vi "getWSIOpenCVIP.vi"(3 "File Path":path=path "C:/Users/vasco/Documents/SVN/fly/scitracks/Trackit studies/OCV im proc/CatWalkLabviewDLL/labview code/notenough.png") -> (0 "Image Dst Out":T1, 1 "return type":i32)   [LabVIEW 2012]
uses:
  <vilib>/vision/Image Controls.llb/IMAQ Image.ctl
  OpenCvGlobals.vi
  <userlib>/OpenCVImProc/CatWalkLabviewDLLd.dll
  <userlib>/OpenCVImProc/CatWalkLabviewDLL.dll
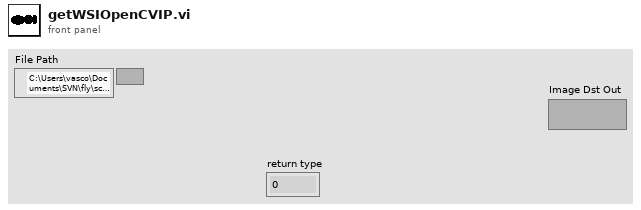
[diagram p1: front panel]
types:
  T1 = typedef "IMAQ Image.ctl" = refnum<image>
  T2 = typedef "Image Type" = u32
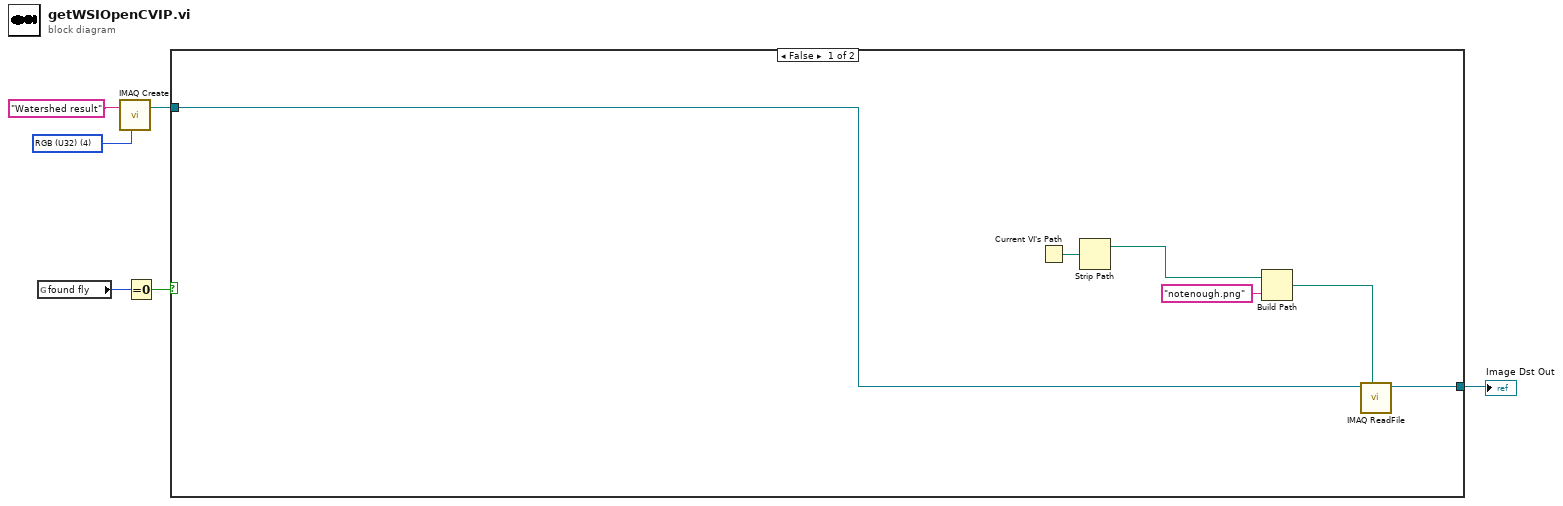
[diagram p0: block diagram]
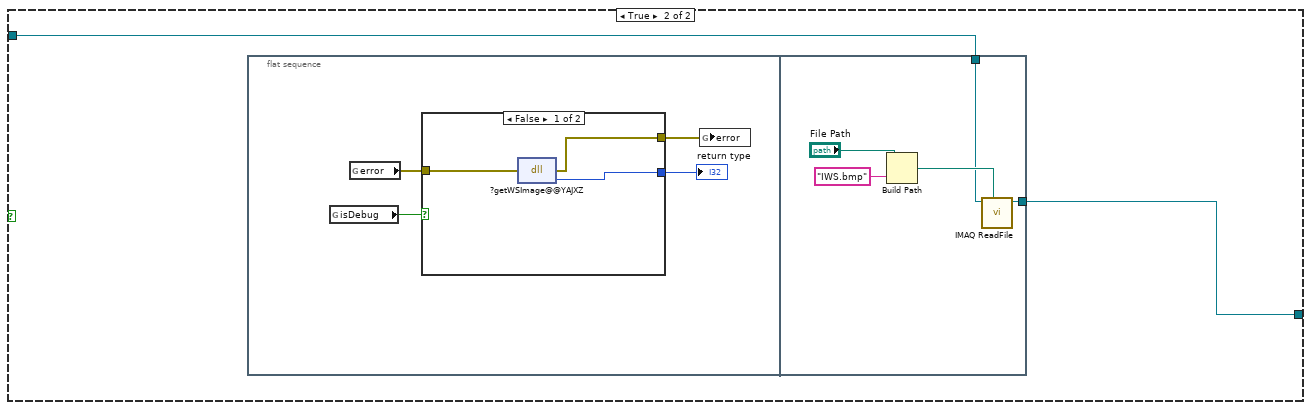
[diagram p2: hidden frame]
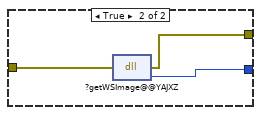
[diagram p3: hidden frame]
diagram:
  w3 = T2 4 items=["Grayscale (U8)", "Grayscale (I16)", "Grayscale (SGL)", "Complex (CSG)", "RGB (U32)", "HSL (U32)", "RGB (U64)", "Grayscale (U16)"] ("Image Type")
  n1 = global read "OpenCvGlobals.vi" "found fly"() -> (w4:i32)
  n2 = call "IMAQ Create"("Image Name"="Watershed result", "Image Type"=w3) -> ("New Image"=w1:T1)  [unwired: 2 in, 2 out]
  n3 = Equal To 0?(x=w4) -> (x = 0?=w5:bool)
  n4 = case shown="False" w5 {
    tunnel: [w12 w13] -> w6
    tunnel: w1 -> [w11 w14]
    frame False {
      n5 = Current VI's Path() -> (path=w8:path)
      n6 = Strip Path(path=w8) -> (stripped path=w7:path)  [unwired: 1 out]
      n7 = Build Path(base path=w7, name or relative path="notenough.png") -> (appended path=w9:path)
      n8 = call "IMAQ ReadFile"("File Path"=w9, "Image"=w11) -> ("Image Out"=w12:T1)  [unwired: 5 in, 4 out]
    }
    frame True {
      n9 = flat-sequence {
        tunnel: w14 -> [w26]
        tunnel: [w25] -> w13
        frame #0 {
          n10 = global read "OpenCvGlobals.vi" "isDebug"() -> (w15:bool)
          n11 = global read "OpenCvGlobals.vi" "error"() -> (w17:errorcluster)
          n12 = case shown="False" w15 {
            tunnel: [w19 w24] -> w18
            tunnel: [w20 w22] -> w16
            tunnel: w17 -> [w21 w23]
            frame False {
              n13 = dll-call lib="C:/Program Files (x86)/National Instruments/LabVIEW 2012/user.lib/OpenCVImProc/CatWalkLabviewDLL.dll" fn="?getWSImage@@YAJXZ"(error in=w21) -> (error out=w20:errorcluster, "return type"=w19:i32)  [unwired: 2 in, 1 out]
            }
            frame True {
              n14 = dll-call lib="C:/Program Files (x86)/National Instruments/LabVIEW 2012/user.lib/OpenCVImProc/CatWalkLabviewDLLd.dll" fn="?getWSImage@@YAJXZ"(error in=w23) -> (error out=w22:errorcluster, "return type"=w24:i32)  [unwired: 2 in, 1 out]
            }
          }
          "return type" <- w18
          n15 = global write "OpenCvGlobals.vi" "error"(w16) -> ()
        }
        frame #1 {
          n16 = Build Path(base path="File Path", name or relative path="IWS.bmp") -> (appended path=w27:path)
          n17 = call "IMAQ ReadFile"("File Path"=w27, "Image"=w26) -> ("Image Out"=w25:T1)  [unwired: 5 in, 4 out]
        }
      }
    }
  }
  "Image Dst Out" <- w6
